vi "PT 100 Temp Convert to R（多项式求值）.vi"(6 "γ":dbl=4.2735e-12 format="%#_6e", 9 "β":dbl=-5.80195e-07 format="%#_6e", 10 "α":dbl=0.00390802 format="%#_6e", 11 "t":dbl) -> (3 "Rt":dbl)   [LabVIEW 2013]
doc: "功能：\n\n计算温度t大于等于0，且小于等于850时的RTD电阻值。"
uses:
  <vilib>/Analysis/polynomials.llb/Scalar Polynomial Evaluation (DBL).vi
  <vilib>/Analysis/NI_AALPro.lvlib
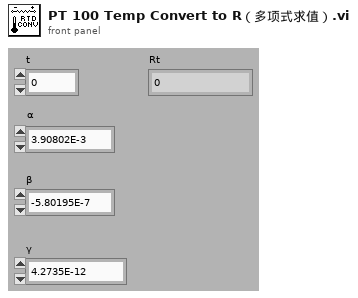
[diagram p1: front panel]
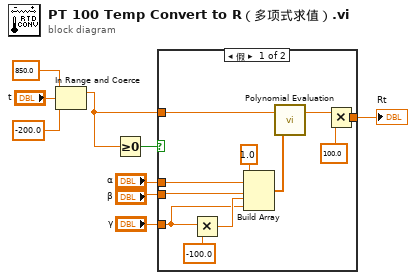
[diagram p0: block diagram]
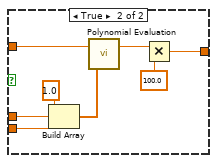
[diagram p2: hidden frame]
diagram:
  n1 = In Range and Coerce(upper limit=850.0 ("上限"), x="t", lower limit=-200.0 ("下限")) -> (coerced(x)=w5:dbl)  [unwired: 1 out]
  n2 = Greater Or Equal To 0?(x=w5) -> (x >= 0?=w6:bool)
  n3 = case shown="假" w6 {
    tunnel: w5 -> [w12 w24]
    tunnel: "α" -> [w19 w27]
    tunnel: "β" -> [w18 w26]
    tunnel: "γ" -> [w16 _]
    tunnel: [w14 w21] -> w1
    frame False {
      n4 = Multiply(x=w16, y=-100.0) -> (x*y=w17:dbl)
      n5 = Build Array(1.0 ("元素"), w19, w18, w17, w16) -> (w13:dbl[])
      n6 = call-poly <vilib>:"Polynomial Evaluation.vi"("P(x)"=w13, "a"=w12) -> ("P(a)"=w11:dbl)  [unwired: 1 out]
      n7 = Multiply(x=w11, y=100.0) -> (x*y=w14:dbl)
    }
    frame True {
      n8 = Build Array(1.0 ("元素"), w27, w26) -> (w25:dbl[])
      n9 = call-poly <vilib>:"Polynomial Evaluation.vi"("P(x)"=w25, "a"=w24) -> ("P(a)"=w23:dbl)  [unwired: 1 out]
      n10 = Multiply(x=w23, y=100.0) -> (x*y=w21:dbl)
    }
  }
  "Rt" <- w1
